vi "Check Dispenser Communication.vi"() -> ()   [LabVIEW 2018]
uses:
  Drivers/EFD Ultimus V/EFD Ultimus V.lvlib
  Controller/Controller.lvclass
panel:
  in  "stop":bool
  in  "on/off":bool
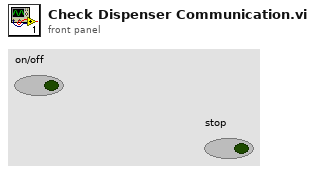
[diagram p1: front panel]
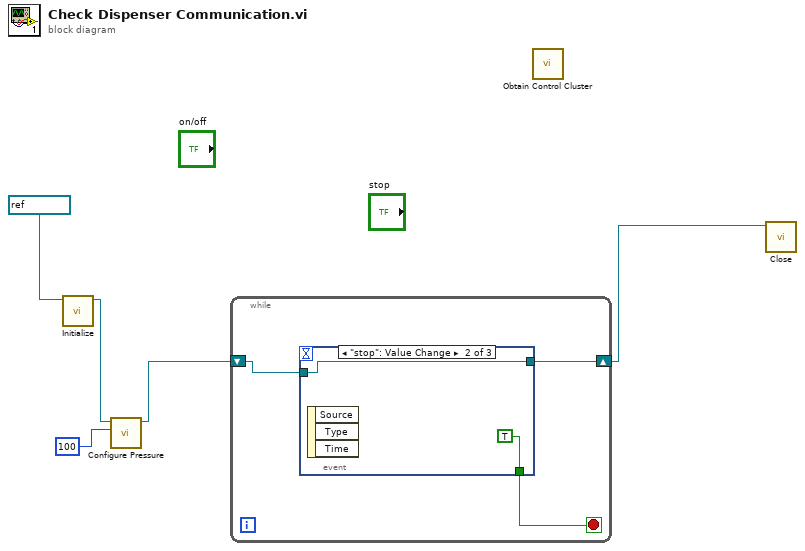
[diagram p0: block diagram]
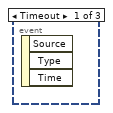
[diagram p2: hidden frame]
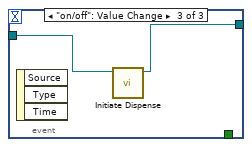
[diagram p3: hidden frame]
diagram:
  n1 = call "Initialize.vi"("VISA resource name"=refnum<visa-resource-name> "COM1") -> ("VISA resource name out"=w4:refnum<visa-resource-name>)  [unwired: 8 in, 1 out]
  n2 = call "Configure Pressure.vi"("Pressure Setting (0000)"=i64 100, "VISA resource name"=w4) -> ("VISA resource name out"=w3:refnum<visa-resource-name>)  [unwired: 8 in, 1 out]
  n3 = while {
    shift-right: [w7] -> w1
    shift-left: w3 -> [w8]
    stop <- w6 stop-if-true
    n4 = event shown="[1] \"stop\": Value Change" {
      selector: _ -> [_ _ _]
      dyn-events: _ -> [_ _ _]
      timeout: _ -> [_ _ _]
      tunnel: w8 -> [_ w9 w12]
      tunnel: [_ w9 w11] -> w7
      tunnel: [_ TRUE _] -> w6
      event Timeout {
        n5 = event-data() -> ()  [unwired: 1 in, 3 out]
      }
      event "stop": Value Change {
        n6 = event-data() -> ()  [unwired: 1 in, 3 out]
      }
      event "on/off": Value Change {
        n7 = event-data() -> ()  [unwired: 1 in, 3 out]
        n8 = call "Initiate Dispense.vi"("VISA resource name"=w12) -> ("VISA resource name out"=w11:refnum<visa-resource-name>)  [unwired: 9 in, 1 out]
      }
    }
  }
  n9 = call "Obtain Control Cluster.vi"() -> ()  [unwired: 11 in, 1 out]
  n10 = call "Close.vi"("VISA resource name"=w1) -> ()  [unwired: 10 in, 1 out]
